vi "TextControlledInstrumCommandsToArrayMulti.vi"(10 "SetGetCommands":string, 11 "Control Array":refnum<vi>[](array[refnum])) -> (2 "Control to Index":T1(c390), 3 "Command Array":string[][](array[string]))   [LabVIEW 2020]
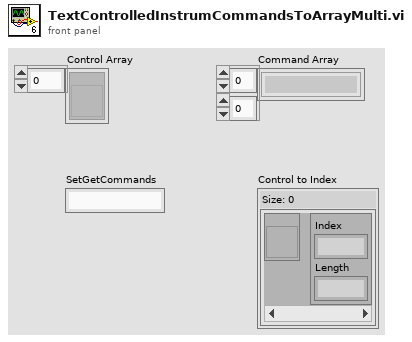
[diagram p1: front panel]
types:
  T1 = map{refnum<vi>, cluster{"Index":i32, "Length":i32}}
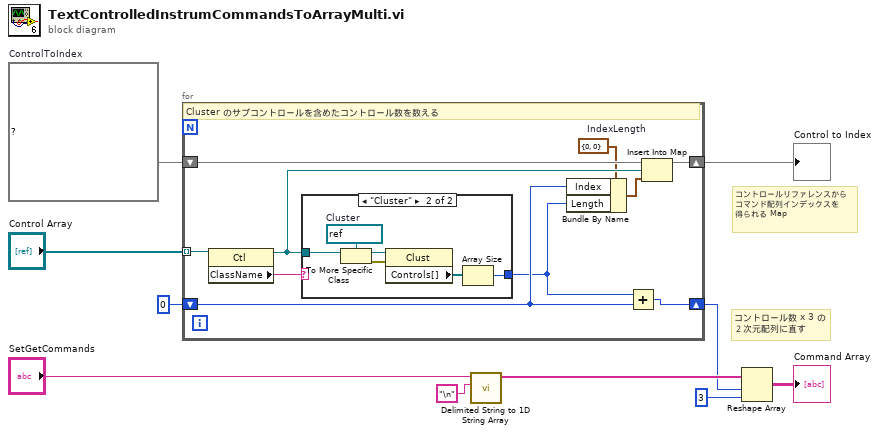
[diagram p0: block diagram]
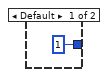
[diagram p2: hidden frame]
diagram:
  w8 = T1 {}  # ControlToIndex
  # "コントロールリファレンスから\nコマンド配列インデックスを\n得られる Map"
  # "コントロール数 x 3 の\n２次元配列に直す"
  n1 = for {
    tunnel: "Control Array" -> [w20] mode=indexing
    shift-right: [w18] -> w3
    shift-left: 0 -> [w13]
    shift-right: [w11] -> w2
    shift-left: w8 -> [w17]
    w14 = cluster{"Index":i32, "Length":i32} {"Index"=0, "Length"=0}  # IndexLength
    # "Cluster のサブコントロールを含めたコントロール数を数える"
    n2 = property class="Ctl"(reference=w20) -> (reference out=w16:refnum<vi>, "ClassName"=w19:string)  [unwired: 1 in, 1 out]
    n3 = case shown="\"Cluster\"" w19 {
      tunnel: w16 -> [_ w27]
      tunnel: [1 w22] -> w12
      frame Default {
      }
      frame "Cluster" {
        w24 = refnum<vi> refnum  # Cluster
        n4 = To More Specific Class(target class=w24, reference=w27) -> (specific class reference=w26:refnum<vi>, error out=w25:errorcluster)  [unwired: 1 in]
        n5 = property class="Clust"(reference=w26, error in=w25) -> ("Controls[]"=w23:refnum<vi>[])  [unwired: 2 out]
        n6 = Array Size(array=w23) -> (size(s)=w22:i32)
      }
    }
    n7 = Bundle By Name(cluster=w14, "Index"=w13, "Length"=w12) -> (w15:cluster{"Index":i32, "Length":i32})
    n8 = Add(x=w12, y=w13) -> (x+y=w18:i32)
    n9 = Insert Into Map(map in=w17, key=w16, value=w15) -> (map out=w11:T1)  [unwired: 2 out]
  }
  "Control to Index" <- w2
  n10 = call <vilib>:"Delimited String to 1D String Array.vi"("delimiter"="\n", "delimited string"="SetGetCommands") -> ("string array"=w6:string[])  [unwired: 9 in]
  n11 = Reshape Array(w6, w3, 3 ("dimension size")) -> (→"Command Array":string[][])
